vi "Calculator.vi"() -> ()   [LabVIEW 2021]
panel:
  out "DIVISION":dbl
  out "MULTIPLICACION":dbl
  out "RESTA":dbl
  in  "stop":bool
  out "SUMA":dbl
  in  "Numeric 2":dbl
  in  "Numeric":dbl
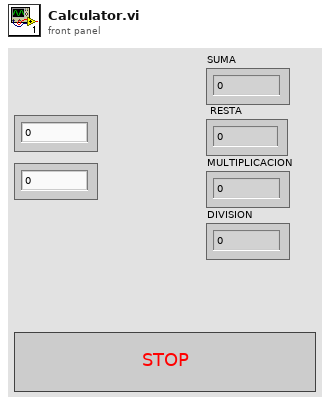
[diagram p1: front panel]
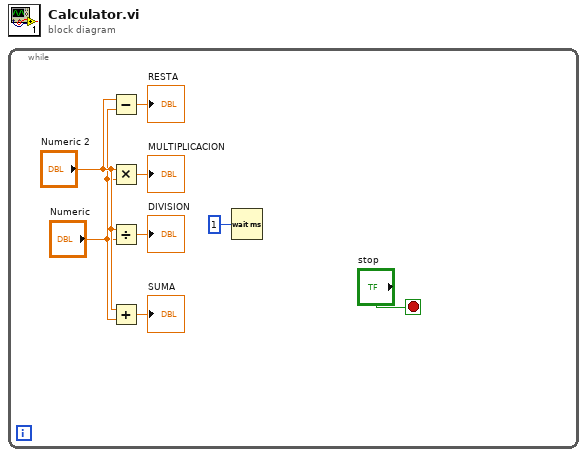
[diagram p0: block diagram]
diagram:
  n1 = while {
    stop <- "stop" stop-if-true
    n2 = Subtract(x="Numeric 2", y="Numeric") -> (x-y=→"RESTA":dbl)
    n3 = Multiply(x="Numeric 2", y="Numeric") -> (x*y=→"MULTIPLICACION":dbl)
    n4 = Divide(x="Numeric 2", y="Numeric") -> (x/y=→"DIVISION":dbl)
    n5 = Add(x="Numeric 2", y="Numeric") -> (x+y=→"SUMA":dbl)
    n6 = Wait (ms)(milliseconds to wait=u32 1) -> ()  [unwired: 1 out]
  }
